vi "Get Tag Info.vi"(8 "error in (no error)":errorcluster, 10 "Tag":string, 11 "TreeControl in":refnum<vi>) -> (0 "error out":errorcluster, 1 "Child Text":string[](array[string]), 2 "Left Cell String":string, 3 "TreeControl out":refnum<vi>, 4 "Child-Only?":bool)   [LabVIEW 2015, in "Shared Variable Custom Device.lvlib"]
uses:
  Shared Variable Custom Device.lvlib
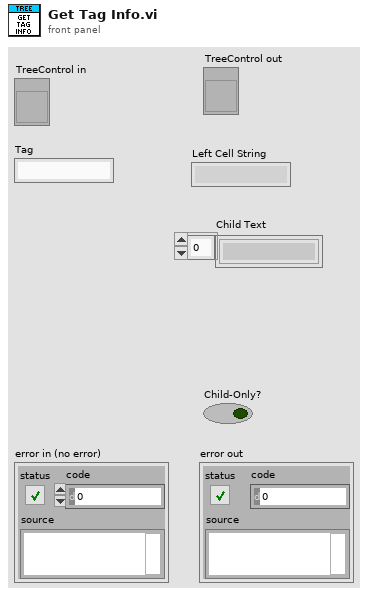
[diagram p1: front panel]
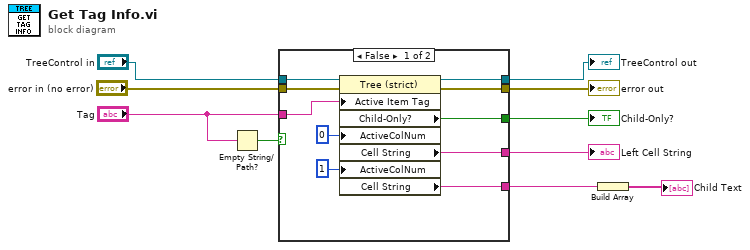
[diagram p0: block diagram]
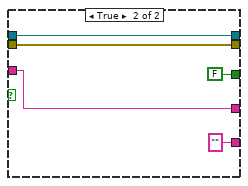
[diagram p2: hidden frame]
diagram:
  n1 = Empty String/Path?(string/path="Tag") -> (empty?=w2:bool)
  n2 = case shown="False" w2 {
    tunnel: [w20 FALSE ("Child-Only?")] -> w10
    tunnel: [w19 w23] -> w9
    tunnel: "Tag" -> [w17 w23]
    tunnel: "TreeControl in" -> [w16 w25]
    tunnel: [w15 w24] -> w7
    tunnel: "error in (no error)" -> [w14 w24]
    tunnel: [w12 w25] -> w5
    tunnel: [w11 "" ("Cell String")] -> w4
    frame False {
      n3 = property class="Tree (strict)"(reference=w16, error in=w14, "Active Item Tag"=w17, "ActiveColNum"=0 ("Active Cell:Active Column Number"), "ActiveColNum"=1 ("Active Cell:Active Column Number")) -> (reference out=w12:refnum<vi>, error out=w15:errorcluster, "Child-Only?"=w20:bool, "Cell String"=w19:string, "Cell String"=w11:string)
    }
    frame True {
    }
  }
  "Child-Only?" <- w10
  "Left Cell String" <- w9
  "error out" <- w7
  "TreeControl out" <- w5
  n4 = Build Array(w4) -> (→"Child Text":string[])
